vi "mhk_Basic Acquisition_XLS wfm.vi"() -> ()   [LabVIEW 2010]
uses:
  <vilib>/Utility/error.llb/DialogType.ctl
  <vilib>/DAQmx/read.llb/DAQmx Read (Analog 1D Wfm NChan NSamp).vi
  <vilib>/DAQmx/create/channels.llb/DAQmx Create Channel (AI-Voltage-Basic).vi
  <vilib>/DAQmx/configure/timing.llb/DAQmx Timing (Sample Clock).vi
  <vilib>/daqmx/miscellaneous.llb/DAQmx Fill In Error Info.vi
  <vilib>/Utility/file.llb/Write To Spreadsheet File (DBL).vi
panel:
  in  "Plot BG Color":bool=TRUE caption="Enable"
  out "# of pts per \nchannel":i32=100
  out "# of channels \nacquired":i32=4
  out "dt (sec)":dbl=9.999999999999999e-05
  in  "Save Data?":bool caption="Enable"
  in  "Maximum Value":dbl=5.0 format="%0.2f"
  in  "Minimum Value":dbl=-5.0 format="%0.2f"
  in  "Physical Channel":tag="Dev1/ai1:4"
  in  "Rate":dbl=10000.0 caption="Sample Rate (Hz)" format="%0.2f"
  in  "Samples per Channel":i32=100
  out "Measurement":waveform(dbl)[](graph)=[{"t0"=timestamp(3409325835.8231497 s since 1904-01-01), "dt"=9.999999999999999e-05, "Y"=[0.08651997436445204, 0.45381023590807823, 0.5951109347819452, 0.7843256935331279, 1.1177404095583972, 1.5958128604998931, 1.7442854091006195, 2.183904538102359, 2.307199316385388, 2.4736777855769523, 2.7779473250526445, 3.2088686788537246, 3.248237556077761, 3.628650776696066, 3.80138554033021, 3.8305307168797875, 3.968626972258675, 4.322336497085482, 4.474623859370708, 4.5605334635456405, 4.67055269020661, 4.67680898464919, 4.653309732352672, 4.691457869197668, 4.873348185674612, 4.814905240028077, 4.729606006042665, 4.736014893032625, 4.651631214331492, 4.598986785485397, 4.470046082949309, 4.3665883358256785, 4.373455000457778, 4.271065401165807, 3.9538254951628162, 3.9532151249732963, 3.838160344248787, 3.58790856654561, 3.3091219824823757, 3.098391674550615, 2.912228766747032, 2.456740012817774, 2.4498733481856747, 2.17307046723838, 1.8645283364360485, 1.5707876827295755, 1.108279671620838, 0.8510086367381817, 0.49974059266945403, 0.3428754539628285, 0.06942960905789361, -0.35782952360606707, -0.6083864864040041, -0.9619434186834315, -1.19556260872219, -1.5744499038666953, -1.8834498123111667, -2.0929593798638875, -2.3972289193395793, -2.6186407055879393, -2.914212469862972, -3.0811487166966764, -3.294473097933897, -3.574785607470931, -3.622241889706107, -3.9071321756645405, -3.9623706778160956, -4.160588396862697, -4.527268288216804, -4.466689046906949, -4.757377849665822, -4.591814935758538, -4.613940855128636, -4.836878566850795, -4.78408154545732, -4.9479659413434245, -4.89791558580279, -4.940641499069185, -4.8593096713156525, -4.836268196661275, -4.488052003540147, -4.510940885647145, -4.475234229560228, -4.256263924069948, -4.150212103640858, -3.9536729026154362, -3.8613544114505447, -3.5601367229224525, -3.2683797723319192, -3.107547227393414, -2.7466658528397474, -2.513504440443129, -2.205877864925077, -2.1050141911069065, -1.8187505722220527, -1.455427716910306, -1.064180425428022, -1.032288583025605, -0.5822931608020264, -0.35843989379558705], "attributes"=variant("NI_ChannelName"=variant(string "Dev1/ai1"), "NI_UnitDescription"=variant(string "Volts"))}, {"t0"=timestamp(3409325835.823163 s since 1904-01-01), "dt"=9.999999999999999e-05, "Y"=[0.4055909909360027, 0.684224982451857, 1.151615955076754, 1.3553270058290352, 1.6893520920438245, 1.9837031159398175, 2.0795312356944486, 2.556535538804285, 2.7416302987762076, 2.8609576708273567, 3.269600512710959, 3.4174626911221657, 3.684804834131901, 3.751792962431715, 3.9262062440870387, 4.304177983947264, 4.2782372508926665, 4.475692007202368, 4.635914181951353, 4.612262337107456, 4.707937864314707, 4.727011932737205, 4.857173375652333, 4.757988219855342, 4.877925962096011, 4.865718558305613, 4.911038544877468, 4.8669392986846525, 4.597918637653737, 4.605700857570116, 4.369335001678518, 4.362773522141179, 4.073915829950865, 4.101687673574022, 3.742790002136296, 3.653218176824244, 3.492690816980499, 3.236335337382122, 2.865840632343516, 2.8176213873714406, 2.60795922727134, 2.1066927091280863, 1.9827875606555376, 1.7909787285988952, 1.5253151036103396, 1.2068544572283089, 0.7315286721396527, 0.5478072450941496, 0.28595843379009367, -0.1879940183721427, -0.47303689687795647, -0.7150486770226142, -0.9504989776299325, -1.4380321665089877, -1.7557298501541185, -1.9943845942564165, -2.0233771782586136, -2.456434827723014, -2.699209570604572, -2.999053926206244, -3.187200537125767, -3.5270241401409956, -3.659779656361583, -3.866847743156224, -4.030121768852809, -4.220404675435652, -4.386425366985076, -4.380626850184637, -4.489730521561327, -4.710379345072787, -4.734336375011444, -4.684133426923429, -4.969023712881863, -4.990539262062441, -4.78225043488876, -4.798883022553179, -4.649800103762932, -4.687490462965789, -4.644459364604633, -4.435254982146672, -4.608294930875576, -4.374370555742058, -4.2866298409985655, -4.006927701651051, -3.726462599566637, -3.5827204199346903, -3.335215308084353, -3.2415234839930416, -3.0033265175328836, -2.7146214178899504, -2.3889889217810603, -2.192297128208258, -2.06472975859859, -1.651203955198828, -1.3280129398480178, -1.0458693197424238, -0.7727286599322489, -0.4617450483718375, -0.3238013855403302, 0.06851405377361369], "attributes"=variant("NI_ChannelName"=variant(string "Dev1/ai2"), "NI_UnitDescription"=variant(string "Volts"))}, {"t0"=timestamp(3409325835.823176 s since 1904-01-01), "dt"=9.999999999999999e-05, "Y"=[0.8616901150547808, 1.2587359233375042, 1.2979522080141606, 1.6563921018097476, 1.9374675740836818, 2.3877681814020204, 2.661671803949095, 2.8234199041718804, 2.9139072847682117, 3.274330881679739, 3.4537797173986022, 3.6909085360271003, 3.7998596148564103, 4.047975096896268, 4.358195745719779, 4.3185216834009825, 4.539780877101962, 4.634083071382793, 4.664448988311411, 4.732505264442884, 4.753563035981323, 4.794000061037019, 4.708548234504227, 4.964293343913083, 4.67802972502823, 4.764549699392681, 4.712210455641347, 4.490340891750847, 4.604480117191076, 4.396801660206916, 4.220557267983032, 4.071169164098025, 4.01562547685171, 3.793908505508591, 3.6385692922757653, 3.3863338114566486, 3.1235694448683127, 3.04605243079928, 2.768791772209845, 2.270271919919431, 2.0041505172887355, 1.9660023804437392, 1.4444410534989471, 1.347544785912656, 0.9315775017548142, 0.7229834894863735, 0.46357615894039733, -0.034180730613116855, -0.18875698110904263, -0.42344431897946105, -0.7776116214484085, -1.0705893124179815, -1.4865565965758232, -1.6913357951597643, -2.151707510605182, -2.1687978759117406, -2.4942777794732507, -2.8432569353312784, -3.0677205725272376, -3.4134952848902858, -3.6146122623371073, -3.7527085177159947, -3.9382610553300577, -3.934446241645558, -4.2864772484511855, -4.372539445173498, -4.345835749382, -4.573503830072939, -4.751884517960143, -4.700155644398327, -4.808496353038118, -4.849543748283334, -4.821619312112796, -4.741813409833064, -4.945371868037965, -4.722586748863185, -4.739371929074984, -4.777214880825221, -4.640339365825373, -4.558244575334941, -4.24436170537431, -4.123813592944121, -4.003570665608692, -3.890194402905362, -3.4333323160496843, -3.4963530381176184, -3.033692434461501, -2.880031739249855, -2.7220984527115695, -2.2682882168034912, -2.1788689840388193, -1.977904599139378, -1.6052735984374522, -1.131168553727836, -1.0943937498092593, -0.6817835016937773, -0.4139835810419019, 0.045930356761375773, 0.1979125339518418, 0.4045228431043428], "attributes"=variant("NI_ChannelName"=variant(string "Dev1/ai3"), "NI_UnitDescription"=variant(string "Volts"))}, {"t0"=timestamp(3409325835.823189 s since 1904-01-01), "dt"=9.999999999999999e-05, "Y"=[1.240577410199286, 1.6922513504440444, 1.717429120761742, 2.056184575945311, 2.275307473982971, 2.556077761162145, 2.93588061159093, 3.0414746543778803, 3.424176763206885, 3.4287545396282844, 3.9062166203802606, 4.007843256935331, 4.2628254036072875, 4.285103915524766, 4.3024994659260845, 4.56434827723014, 4.610583819086276, 4.56572161015656, 4.7372356334116645, 4.78133487960448, 4.720908230842006, 4.868617816705832, 4.851832636494033, 4.7811822870571, 4.870143742179632, 4.7373882259590445, 4.7048860133671075, 4.625843073824274, 4.34690389721366, 4.34919278542436, 4.062013611255226, 3.904385509811701, 3.739432966093936, 3.501388592181158, 3.1800286873989076, 3.119296853541673, 2.7201147495956297, 2.698446607867672, 2.3937192907498397, 2.0725119785149695, 1.7316202276680808, 1.5356913968321788, 1.099276711325419, 0.9488204596087527, 0.6703390606402784, 0.3827021088290048, 0.039063692129276406, -0.40116580706198307, -0.630054628131962, -0.9326456495864742, -1.2158574175237282, -1.6771446882534258, -1.9157994323557237, -2.0419934690389723, -2.28385265663625, -2.5467696157719657, -2.9309976500747705, -3.053682058168279, -3.2883693960386973, -3.663136692403943, -3.833124790185247, -4.069643238624225, -4.076052125614185, -4.381542405468917, -4.412213507492294, -4.401989806817835, -4.6333201086458935, -4.67452009643849, -4.804376354258858, -4.788506729331339, -4.900814844203009, -4.949186681722464, -4.708700827051607, -4.808496353038118, -4.88799707022309, -4.659871211890011, -4.698782311471907, -4.494918668172247, -4.4875942258980075, -4.2220831934568315, -3.9387188329721976, -3.848078859828486, -3.58699301126133, -3.6228522598956268, -3.292641987365337, -2.9454939420758692, -2.7793206579790644, -2.533341471602527, -2.434766685995056, -2.053895687734611, -1.673024689474166, -1.3179418317209388, -1.1598559526352732, -0.836970122379223, -0.5011139255958739, -0.24185918759727776, -0.09186071352275155, 0.3357036042359691, 0.6701864680928984, 1.0193182164983061], "attributes"=variant("NI_ChannelName"=variant(string "Dev1/ai4"), "NI_UnitDescription"=variant(string "Volts"))}]
  # "Channel Parameters"
  # "Timing Parameters"
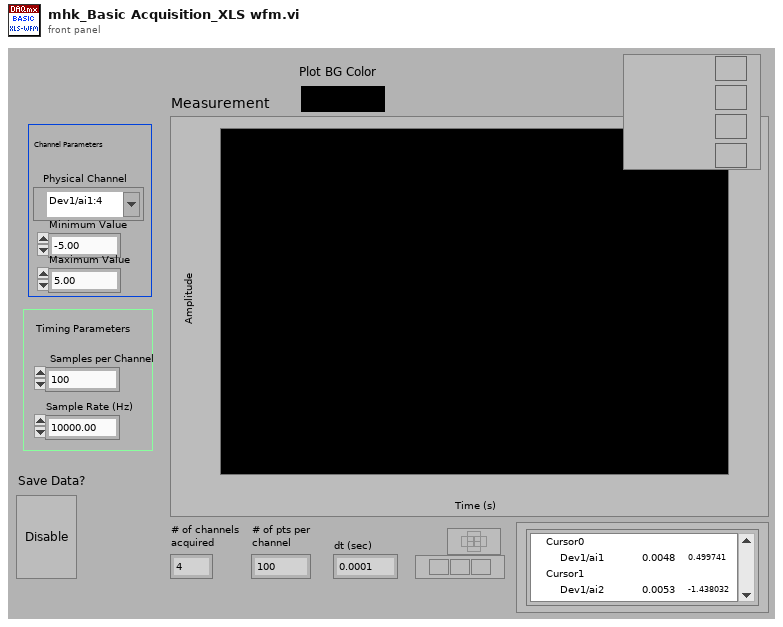
[diagram p1: front panel]
types:
  T1 = typedef "DialogType.ctl" = u16
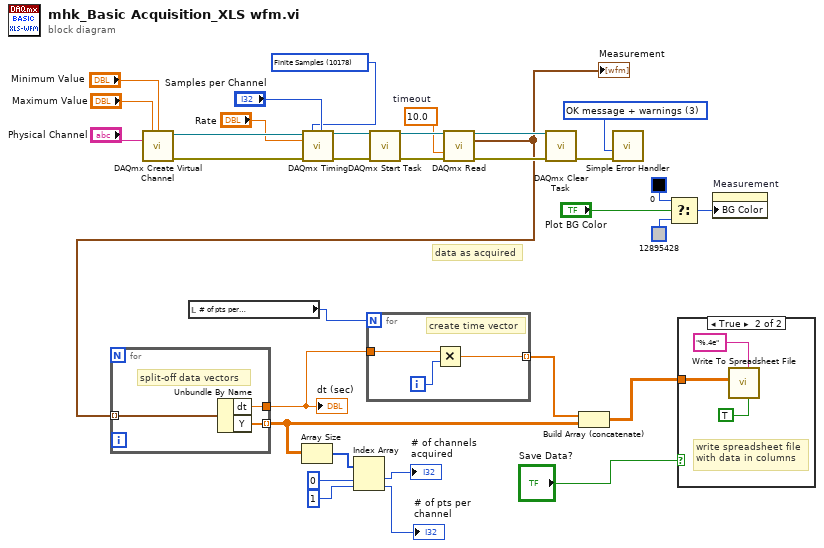
[diagram p0: block diagram]
diagram:
  w18 = T1 3 items=["no dialog", "OK message", "continue or stop message", "OK message + warnings", "continue/stop + warnings"] ("type of dialog (OK msg:1)")
  w19 = 10.0  # timeout
  w23 = 10178 items=["Finite Samples"=10178, "Continuous Samples"=10123] ("sample mode")
  # "data as acquired"
  n1 = call-poly <vilib>:"DAQmx Create Virtual Channel.vi"("maximum value"="Maximum Value", "minimum value"="Minimum Value", "physical channels"="Physical Channel") -> ("task out"=w27:refnum<k21>, "error out"=w31:errorcluster)  [unwired: 11 in]
  n2 = local read "# of pts per \nchannel"() -> (w6:i32)
  n3 = call-poly <vilib>:"DAQmx Timing.vi"("task/channels in"=w27, "sample mode"=w23, "samples per channel"="Samples per Channel", "rate"="Rate", "error in"=w31) -> ("task out"=w22:refnum<k21>, "error out"=w21:errorcluster)  [unwired: 9 in]
  n4 = call <vilib>:"DAQmx Start Task.vi"("task/channels in"=w22, "error in"=w21) -> ("task out"=w26:refnum<k21>, "error out"=w30:errorcluster)  [unwired: 12 in]
  n5 = call-poly <vilib>:"DAQmx Read.vi"("task/channels in"=w26, "timeout"=w19, "error in"=w30) -> ("task out"=w25:refnum<k21>, "data"=w13:waveform(dbl)[], "error out"=w20:errorcluster)  [unwired: 10 in]
  "Measurement" <- w13
  n6 = for {
    tunnel: [w36] -> w12
    tunnel: [w35] -> w10 mode=indexing
    tunnel: w13 -> [w34] mode=indexing
    # "split-off data vectors"
    n7 = Unbundle By Name(w34) -> ("dt"=w36:dbl, "Y"=w35:dbl[])
  }
  "dt (sec)" <- w12
  n8 = Array Size(array=w10) -> (size(s)=w9:i32[])
  n9 = Index Array(array=w9, index #1=0 ("index"), index #2=1 ("index")) -> (element #1=→"# of channels \nacquired":i32, element #2=→"# of pts per \nchannel":i32)
  n10 = for {
    N: w6 -> [_]
    tunnel: [w38] -> w11 mode=indexing
    tunnel: w12 -> [w37]
    i -> [w39]
    # "create time vector"
    n11 = Multiply(x=w37, y=w39) -> (x*y=w38:dbl)
  }
  n12 = call <vilib>:"DAQmx Clear Task.vi"("task in"=w25, "error in"=w20) -> ("error out"=w28:errorcluster)  [unwired: 13 in]
  n13 = Build Array (concatenate)(w11, w10) -> (w5:dbl[][])
  n14 = call <vilib>:"Simple Error Handler.vi"("type of dialog (OK msg:1)"=w18, "error in (no error)"=w28) -> ()  [unwired: 3 in, 5 out]
  n15 = Select(t=u32 0, s="Plot BG Color", f=u32 12895428) -> (s? t:f=w4:u32)
  n16 = case shown="True" "Save Data?" {
    tunnel: w5 -> [_ w40]
    frame False {
    }
    frame True {
      # "write spreadsheet file\nwith data in columns"
      n17 = call-poly <vilib>:"Write To Spreadsheet File.vi"("transpose? (no:F)"=TRUE, "format (%.3f)"="%.4e", "2D data"=w40) -> ()  [unwired: 5 in, 1 out]
    }
  }
  n18 = property on="Measurement" class="WFGraph (strict)"("BG Color"=w4) -> ()  [unwired: 2 in, 2 out]
